vi "testing-turning.vi"() -> ()   [LabVIEW 2015]
uses:
  <vilib>/FPGAPlugInAG/myRIO-1900/niLvFpga_Open_myRIO-1900.vi
  <vilib>/rvi/interface/common/dynamic/niFpgaDynamicAddResources.vi
  <vilib>/Utility/error.llb/Error Cluster From Error Code.vi
  <vilib>/rvi/errors/niLvFpgaAdjustHostInterfaceError.vi
  <vilib>/FPGAPlugInAG/Dynamic/niLvFpga_Close_Dynamic.vi
  <vilib>/rvi/interface/nirviOpenFPGA/nirviOpenFPGA.xnode
  FPGA Bitfiles/Milestone4_FPGATarget_FPGA_pNQ72xw5+dw.lvbitx
  FPGA.vi
  <vilib>/rvi/interface/nirviReadWriteControl/nirviReadWriteControl.xnode
  <vilib>/rvi/interface/nirviCloseFPGA/nirviCloseFPGA.xnode
  class/Car.lvclass
  NiFpgaLv.dll
  <vilib>/rvi/interface/Simulation/niFpgaSimulationCallBeginRW.vi
panel:
  in  "pwm multi":i16
  in  "Wheel Angle 2":dbl
  in  "Wheel Angle":dbl
  in  "speed":dbl=50.0 format="%#_13g"
  in  "Turn time":i32=10
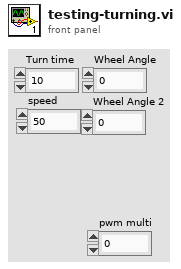
[diagram p1: front panel]
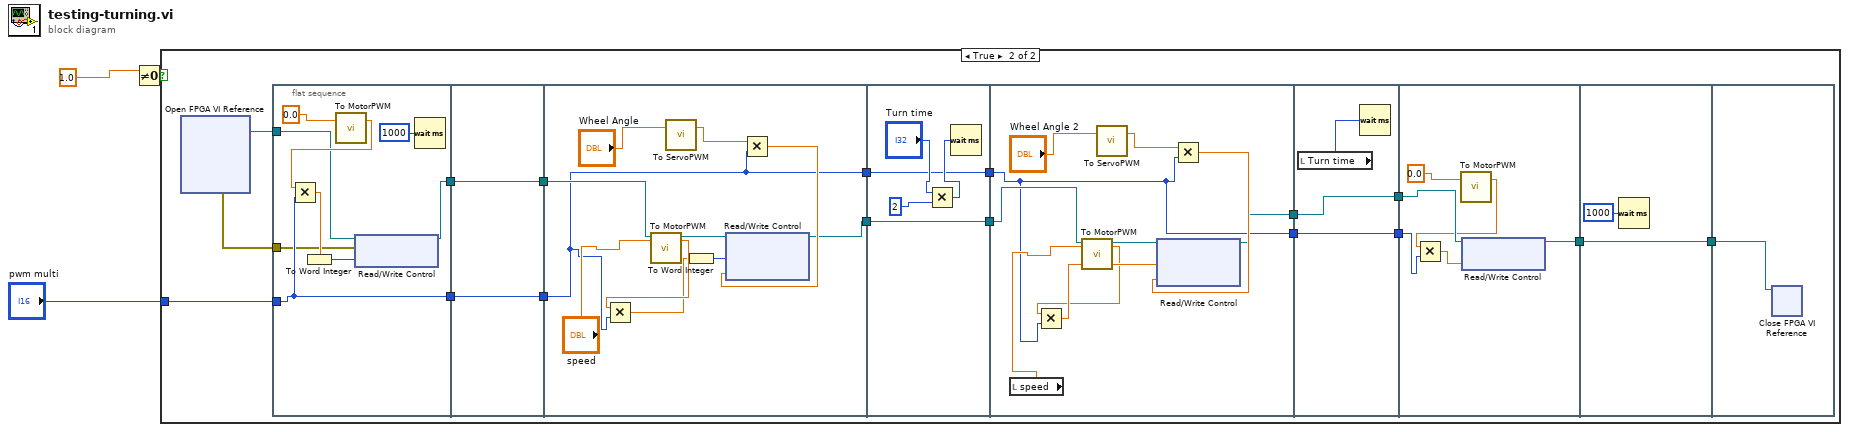
[diagram p0: block diagram]
diagram:
  n1 = Not Equal To 0?(x=1.0) -> (x != 0?=w3:bool)
  n2 = case shown="True" w3 {
    tunnel: "pwm multi" -> [_ w11]
    frame False {
    }
    frame True {
      n3 = xnode "Open FPGA VI Reference"() -> ("FPGA VI Reference Out"=w20:refnum<k20>, "error out"=w4:errorcluster)  [unwired: 2 in]
      n4 = flat-sequence {
        tunnel: w20 -> [w27]
        tunnel: [w22] -> w19
        tunnel: w11 -> [w24]
        tunnel: [w24] -> w10
        tunnel: w4 -> [w23]
        tunnel: w19 -> [w31]
        tunnel: [w31] -> w18
        tunnel: w10 -> [w30]
        tunnel: [w30] -> w9
        tunnel: w18 -> [w36]
        tunnel: [w32] -> w17
        tunnel: w9 -> [w35]
        tunnel: [w35] -> w7
        tunnel: w17 -> [w43]
        tunnel: [w43] -> w16
        tunnel: [w42] -> w8
        tunnel: w7 -> [w42]
        tunnel: w16 -> [w49]
        tunnel: [w47] -> w15
        tunnel: w8 -> [w48]
        tunnel: [w48] -> w6
        tunnel: w15 -> [w57]
        tunnel: [w57] -> w14
        tunnel: w6 -> [w56]
        tunnel: [w56] -> w5
        tunnel: w14 -> [w62]
        tunnel: [w60] -> w13
        tunnel: w5 -> [w59]
        tunnel: w13 -> [w65]
        tunnel: [w65] -> w12
        tunnel: w12 -> [w67]
        frame #0 {
          n5 = call "To MotorPWM.vi"("Speed"=0.0) -> ("MotorPWM"=w28:dbl)  [unwired: 1 in, 1 out]
          n6 = Multiply(x=w28, y=w24) -> (x*y=w25:dbl)
          n7 = To Word Integer(number=w25) -> (16bit integer=w26:i16)
          n8 = xnode "Read/Write Control"("FPGA VI Reference In"=w27, "error in"=w23, "Motor PWM"=w26) -> ("FPGA VI Reference Out"=w22:refnum<k20>)  [unwired: 1 out]
          n9 = Wait (ms)(milliseconds to wait=1000) -> ()  [unwired: 1 out]
        }
        frame #1 {
        }
        frame #2 {
          n10 = call "To MotorPWM.vi"("Speed"="speed") -> ("MotorPWM"=w40:dbl)  [unwired: 1 in, 1 out]
          n11 = Multiply(x=w40, y=w35) -> (x*y=w33:dbl)
          n12 = call "To ServoPWM.vi"("Wheel Angle"="Wheel Angle") -> ("ServoPWM"=w38:dbl)  [unwired: 1 in, 1 out]
          n13 = To Word Integer(number=w33) -> (16bit integer=w34:i16)
          n14 = Multiply(x=w38, y=w35) -> (x*y=w37:dbl)
          n15 = xnode "Read/Write Control"("FPGA VI Reference In"=w36, "Motor PWM"=w34, "Servo PWM"=w37) -> ("FPGA VI Reference Out"=w32:refnum<k20>)  [unwired: 1 in, 1 out]
        }
        frame #3 {
          n16 = Multiply(x="Turn time", y=2) -> (x*y=w44:i32)
          n17 = Wait (ms)(milliseconds to wait=w44) -> ()  [unwired: 1 out]
        }
        frame #4 {
          n18 = local read "speed"() -> (w50:dbl)
          n19 = call "To MotorPWM.vi"("Speed"=w50) -> ("MotorPWM"=w53:dbl)  [unwired: 1 in, 1 out]
          n20 = Multiply(x=w53, y=w48) -> (x*y=w54:dbl)
          n21 = call "To ServoPWM.vi"("Wheel Angle"="Wheel Angle 2") -> ("ServoPWM"=w52:dbl)  [unwired: 1 in, 1 out]
          n22 = Multiply(x=w52, y=w48) -> (x*y=w51:dbl)
          n23 = xnode "Read/Write Control"("FPGA VI Reference In"=w49, "Motor PWM"=w54, "Servo PWM"=w51) -> ("FPGA VI Reference Out"=w47:refnum<k20>)  [unwired: 1 in, 1 out]
        }
        frame #5 {
          n24 = local read "Turn time"() -> (w58:i32)
          n25 = Wait (ms)(milliseconds to wait=w58) -> ()  [unwired: 1 out]
        }
        frame #6 {
          n26 = call "To MotorPWM.vi"("Speed"=0.0) -> ("MotorPWM"=w61:dbl)  [unwired: 1 in, 1 out]
          n27 = Multiply(x=w61, y=w59) -> (x*y=w63:dbl)
          n28 = xnode "Read/Write Control"("FPGA VI Reference In"=w62, "Motor PWM"=w63) -> ("FPGA VI Reference Out"=w60:refnum<k20>)  [unwired: 1 in, 1 out]
        }
        frame #7 {
          n29 = Wait (ms)(milliseconds to wait=1000) -> ()  [unwired: 1 out]
        }
        frame #8 {
          n30 = xnode "Close FPGA VI Reference"("FPGA VI Reference In"=w67) -> ()  [unwired: 1 in, 1 out]
        }
      }
    }
  }
